vi "aryth_mux.vi"(2 "Control":T3, 3 "Flags_input":T1, 4 "Results_input":T2) -> (0 "Flags":T4, 1 "Result":T5)   [LabVIEW 2013]
panel:
  # "R1"
  # "R1"
  # "R1"
  # "R1"
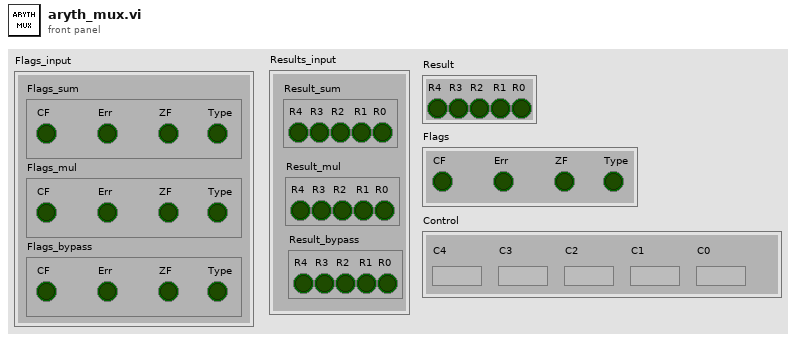
[diagram p1: front panel]
types:
  T1 = cluster{"Flags_sum":cluster{"CF":bool, "Err":bool, "ZF":bool, "Type":bool}, "Flags_mul":cluster{"CF":bool, "Err":bool, "ZF":bool, "Type":bool}, "Flags_bypass":cluster{"CF":bool, "Err":bool, "ZF":bool, "Type":bool}}
  T2 = cluster{"Result_sum":cluster{"R4":bool, "R3":bool, "R2":bool, bool, "R0":bool}, "Result_mul":cluster{"R4":bool, "R3":bool, "R2":bool, bool, "R0":bool}, "Result_bypass":cluster{"R4":bool, "R3":bool, "R2":bool, bool, "R0":bool}}
  T3 = cluster{"C4":bool, "C3":bool, "C2":bool, "C1":bool, "C0":bool}
  T4 = cluster{"CF":bool, "Err":bool, "ZF":bool, "Type":bool}
  T5 = cluster{"R4":bool, "R3":bool, "R2":bool, bool, "R0":bool}
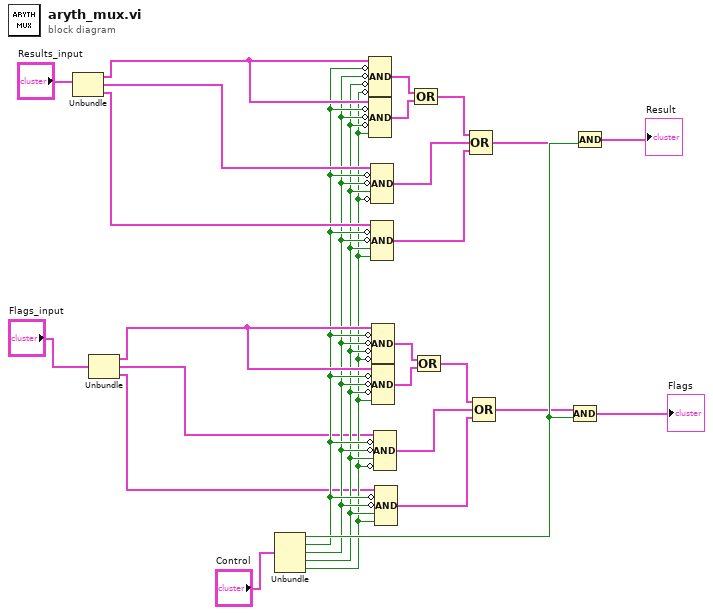
[diagram p0: block diagram]
diagram:
  n1 = Unbundle("Results_input") -> ("Result_sum"=w15:T5, "Result_mul"=w13:T5, "Result_bypass"=w14:T5)
  n2 = Unbundle("Flags_input") -> ("Flags_sum"=w10:T4, "Flags_mul"=w2:T4, "Flags_bypass"=w3:T4)
  n3 = Unbundle("Control") -> ("C4"=w28:bool, "C3"=w9:bool, "C2"=w8:bool, "C1"=w7:bool, "C0"=w6:bool)
  n4 = Compound Arithmetic op=AND(w15, invert w9, invert w8, invert w7, invert w6) -> (w24:T5)
  n5 = Compound Arithmetic op=AND(w15, invert w9, invert w8, invert w7, w6) -> (w23:T5)
  n6 = Compound Arithmetic op=AND(w13, invert w9, invert w8, w7, invert w6) -> (w11:T5)
  n7 = Compound Arithmetic op=AND(w14, invert w9, invert w8, w7, w6) -> (w12:T5)
  n8 = Compound Arithmetic op=AND(w10, invert w9, invert w8, invert w7, invert w6) -> (w21:T4)
  n9 = Compound Arithmetic op=AND(w10, invert w9, invert w8, invert w7, w6) -> (w20:T4)
  n10 = Compound Arithmetic op=AND(w2, invert w9, invert w8, w7, invert w6) -> (w4:T4)
  n11 = Compound Arithmetic op=AND(w3, invert w9, invert w8, w7, w6) -> (w5:T4)
  n12 = Compound Arithmetic op=OR(w24, w23) -> (w22:T5)
  n13 = Compound Arithmetic op=OR(w21, w20) -> (w19:T4)
  n14 = Compound Arithmetic op=OR(w22, w11, w12) -> (w17:T5)
  n15 = Compound Arithmetic op=OR(w19, w4, w5) -> (w18:T4)
  n16 = Compound Arithmetic op=AND(w18, w28) -> (→"Flags":T4)
  n17 = Compound Arithmetic op=AND(w17, w28) -> (→"Result":T5)
